vi "Cleanup Server.vi"(8 "error in (no error)":errorcluster, 11 "TCPMessaging in":refnum<class "TCPMessaging.lvclass">) -> (0 "error out":errorcluster)   [LabVIEW 2020, in "Vecto.lvlib" / "TCPMessaging.lvclass"]
uses:
  TCPMessaging.lvclass
  TCPMessaging.lvclass/TCPMessaging.ctl
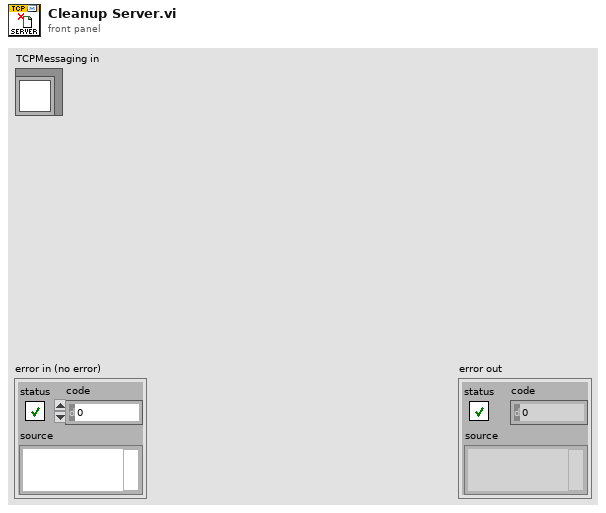
[diagram p1: front panel]
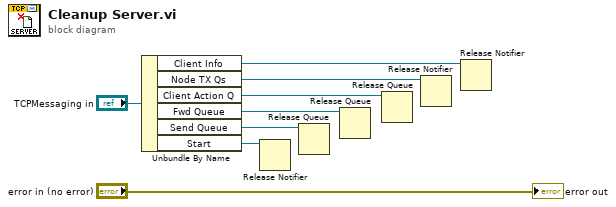
[diagram p0: block diagram]
diagram:
  n1 = Unbundle By Name("TCPMessaging in") -> ("Client Info"=w5:refnum<notifier>, "Node TX Qs"=w4:refnum<notifier>, "Client Action Q"=w1:refnum<queue>, "Fwd Queue"=w2:refnum<queue>, "Send Queue"=w3:refnum<queue>, "Start"=w6:refnum<notifier>)
  n2 = Release Notifier(notifier=w6) -> ()  [unwired: 2 in, 3 out]
  n3 = Release Queue(queue=w3) -> ()  [unwired: 2 in, 3 out]
  n4 = Release Queue(queue=w2) -> ()  [unwired: 2 in, 3 out]
  n5 = Release Queue(queue=w1) -> ()  [unwired: 2 in, 3 out]
  n6 = Release Notifier(notifier=w4) -> ()  [unwired: 2 in, 3 out]
  n7 = Release Notifier(notifier=w5) -> ()  [unwired: 2 in, 3 out]
  "error out" <- "error in (no error)"
